vi "acc_gyro_sync_logger.vi"() -> ()   [LabVIEW 2012]
uses:
  acc_gyro_sync_data.ctl
  <vilib>/Instr/_visa.llb/VISA Configure Serial Port (Instr).vi
panel:
  out "Error":u32(graph)
  out "rate":dbl[unit]
  out "errors":i32
  out "trigger":bool
  in  "frame rate (fps)":dbl=100.0
  in  "Baud rate":u32=57600
  out "Accelerometer":waveform(dbl)[](graph)
  out "Gyro":waveform(dbl)[](graph)
  in  "accel range (m/s2)":dbl(ring)=2.0 items=["2"=2.0, "4"=4.0, "8"=8.0, "16"=16.0]
  in  "gyro range (deg/s)":dbl(ring)=250.0 items=["250"=250.0, "500"=500.0, "1000"=1000.0, "2000"=2000.0]
  in  "Serial port":refnum<visa-resource-name>="COM3"
  in  "stop":bool
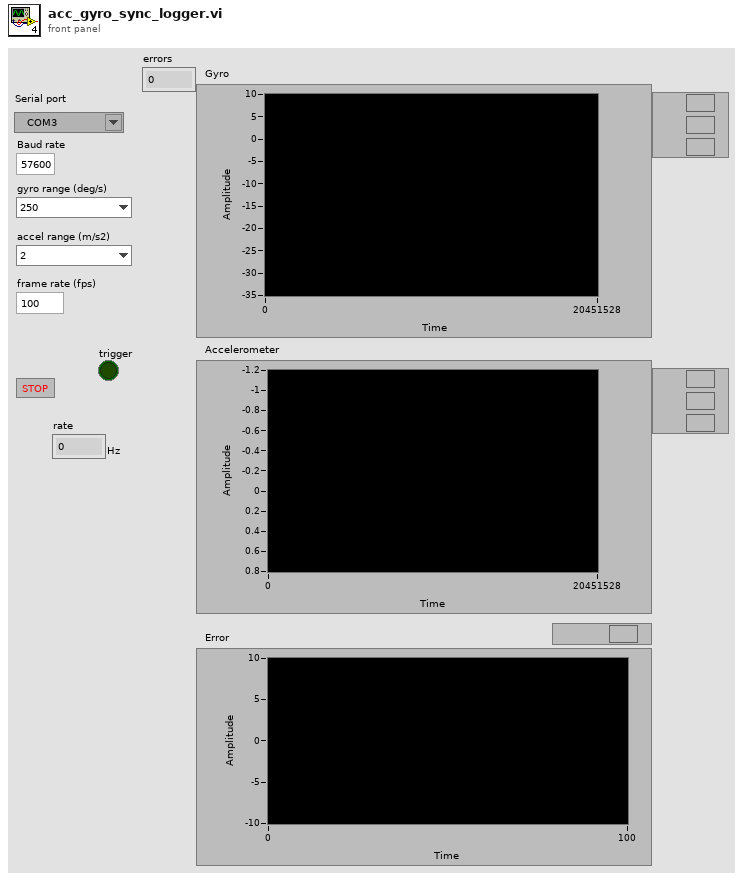
[diagram p1: front panel]
types:
  T1 = typedef "acc_gyro_sync_data.ctl" = cluster{"microsec":u32, "istrigger":u8, "gyro_x":dbl, "gyro_y":dbl, "gyro_z":dbl, "acc_x":dbl, "acc_y":dbl, "acc_z":dbl, "error":u32}
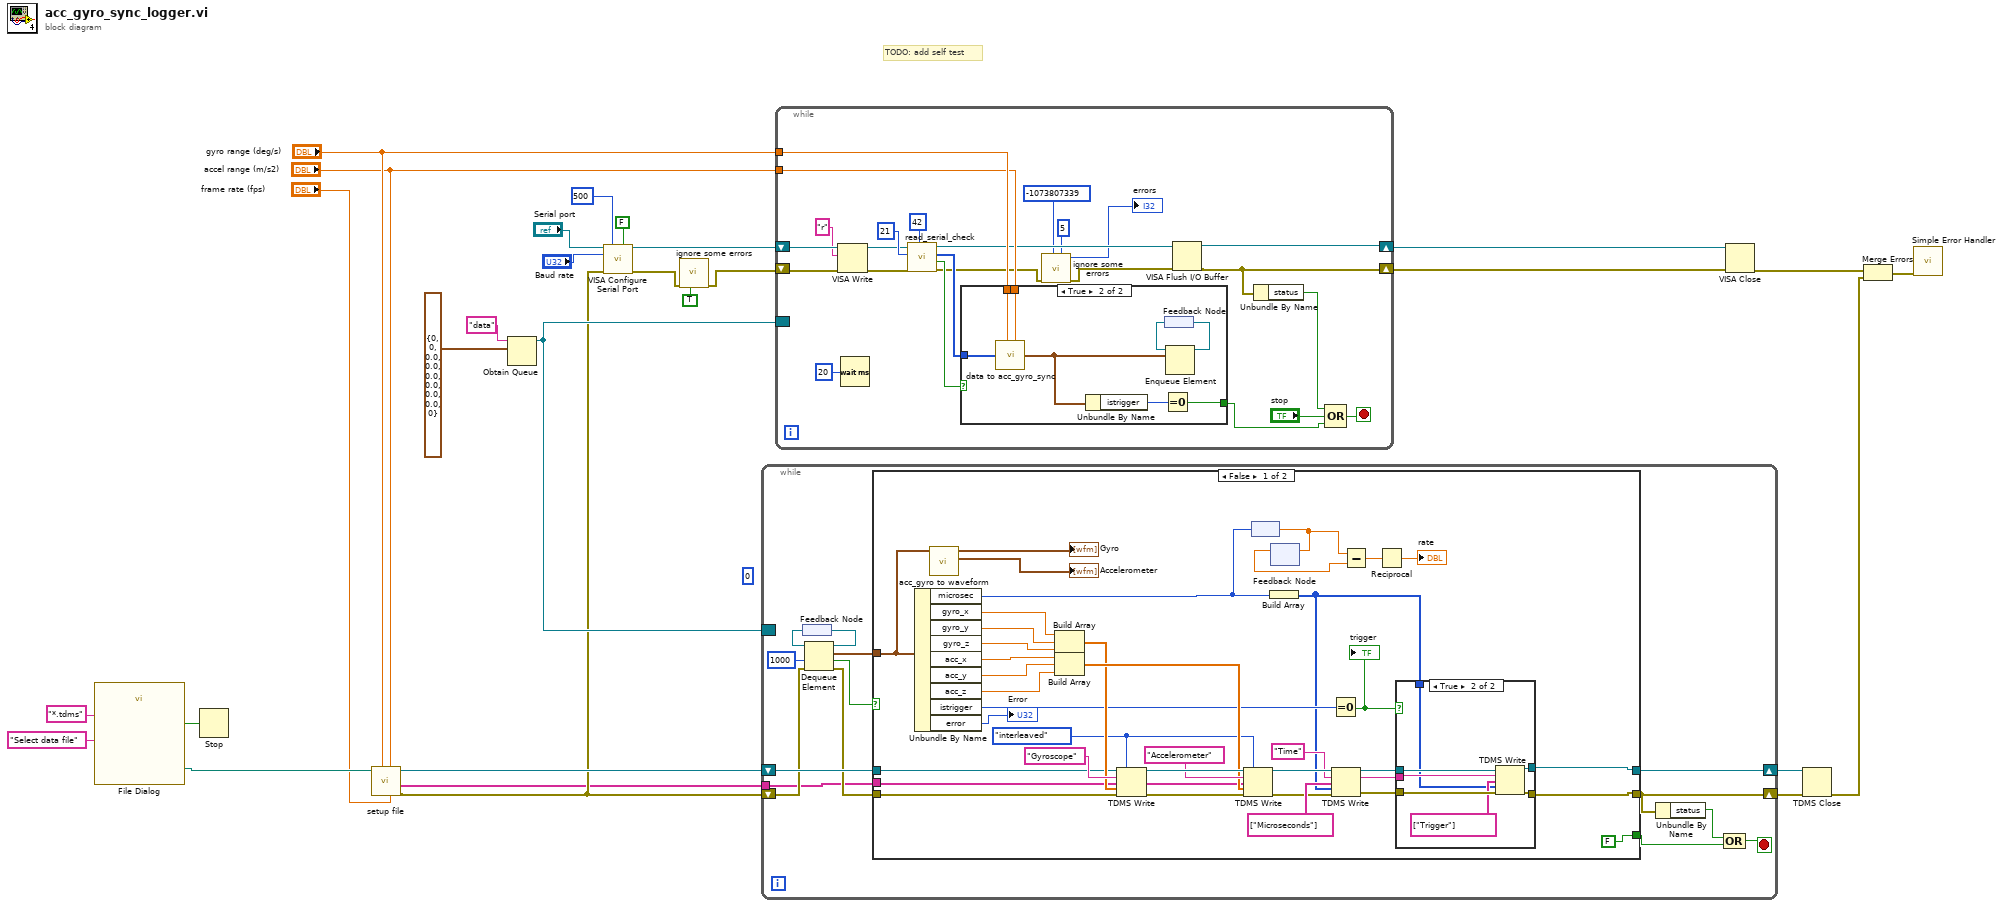
[diagram p0: block diagram]
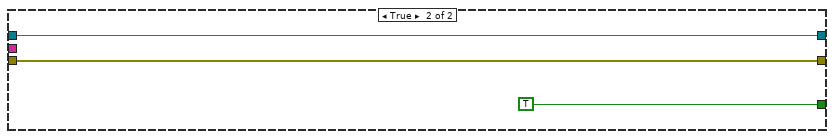
[diagram p3: hidden frame]
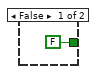
[diagram p4: hidden frame]
diagram:
  (unwired) u64 0 ("milliseconds")
  # "TODO: add self test"
  n1 = call "File Dialog"("prompt"="Select data file", "pattern (all files)"="*.tdms") -> ("selected path"=w21:path, "cancelled"=w20:bool)  [unwired: 10 in, 2 out]
  n2 = Stop(stop? (T)=w20) -> ()
  n3 = call "setup file.vi"("frame rate"="frame rate (fps)", "accel range"="accel range (m/s2)", "gyro range"="gyro range (deg/s)", "selected path"=w21) -> ("error out"=w10:errorcluster, "channel names"=w7:string[], "tdms file out"=w11:refnum<k34>)  [unwired: 5 in]
  n4 = Obtain Queue(name (unnamed)="data", element data type=T1 {"microsec"=0, "istrigger"=0, "gyro_x"=0.0, "gyro_y"=0.0, "gyro_z"=0.0, "acc_x"=0.0, "acc_y"=0.0, "acc_z"=0.0, "error"=0} ("acc gyro data")) -> (queue out=w19:refnum<queue>)  [unwired: 3 in, 2 out]
  n5 = call-poly "VISA Configure Serial Port"("VISA resource name"="Serial port", "timeout (10sec)"=u32 500, "Enable Termination\nChar (T)"=FALSE ("Enable Termination\nChar (T)"), "baud rate (9600)"="Baud rate", "error in (no error)"=w10) -> ("VISA resource name out"=w5:refnum<visa-resource-name>, "error out"=w4:errorcluster)  [unwired: 9 in]
  n6 = call "ignore some errors.vi"("reset"=TRUE, "error in"=w4) -> ("error out"=w3:errorcluster)  [unwired: 8 in, 1 out]
  n7 = while {
    border: w19 -> [_]
    shift-right: [w33] -> w16
    shift-left: w10 -> [w36]
    shift-right: [w38] -> w15
    shift-left: w11 -> [w39]
    tunnel: w7 -> [w29]
    stop <- w30 stop-if-true
    n8 = feedback #1() -> (w42:refnum<queue>)
    n9 = Dequeue Element(queue=w42, timeout in ms (-1)=1000, error in (no error)=w36) -> (queue out=w41:refnum<queue>, element=w40:T1, timed out?=w34:bool, error out=w35:errorcluster)
    n10 = feedback-in #1(w41) -> ()
    n11 = case shown="False" w34 {
      tunnel: w40 -> [w67 _]
      tunnel: [w50 w91] -> w33
      tunnel: w39 -> [w58 w92]
      tunnel: [w51 w92] -> w38
      tunnel: w35 -> [w59 w91]
      tunnel: [FALSE TRUE] -> w31
      tunnel: w29 -> [w64 _]
      frame False {
        w57 = enum16{"decimated", "interleaved"}."interleaved" ("data layout (0:decimated)")
        n12 = Unbundle By Name(w67) -> ("microsec"=w48:u32, "gyro_x"=w81:dbl, "gyro_y"=w80:dbl, "gyro_z"=w79:dbl, "acc_x"=w78:dbl, "acc_y"=w77:dbl, "acc_z"=w76:dbl, "istrigger"=w52:u8, "error"=→"Error":u32)
        n13 = call "acc_gyro to waveform.vi"("acc gyro data"=w67) -> ("accel plot"=→"Accelerometer":waveform(dbl)[], "gyro plot"=→"Gyro":waveform(dbl)[])  [unwired: 9 in]
        n14 = Build Array(w81, w80, w79) -> (w68:dbl[])
        n15 = Build Array(w78, w77, w76) -> (w71:dbl[])
        n16 = TDMS Write(0:w58, 1:w57, 5:"Gyroscope" ("group name (Untitled)"), 7:w64, 9:w68, 11:w59) -> (4:w74:refnum<k34>, 8:w63:string[], 15:w73:errorcluster)  [unwired: 1 out]
        n17 = TDMS Write(0:w74, 1:w57, 5:"Accelerometer" ("group name (Untitled)"), 7:w63, 9:w71, 11:w73) -> (4:w62:refnum<k34>, 15:w61:errorcluster)  [unwired: 2 out]
        n18 = node(w48) -> (w47:dbl[unit])
        n19 = Build Array(w48) -> (w49:u32[])
        n20 = feedback-in #2(w47) -> ()
        n21 = feedback #2() -> (w46:dbl[unit])  [unwired: 1 in]
        n22 = Equal To 0?(x=w52) -> (x = 0?=w56:bool)
        "trigger" <- w56
        n23 = TDMS Write(0:w62, 5:"Time" ("group name (Untitled)"), 7:string[] ["Microseconds"] ("channel name(s) in (Untitled)"), 9:w49, 11:w61) -> (4:w55:refnum<k34>, 6:w54:string, 15:w53:errorcluster)  [unwired: 1 in, 1 out]
        n24 = Subtract(x=w47, y=w46) -> (x-y=w45:dbl[unit])
        n25 = Reciprocal(x=w45) -> (1/x=→"rate":dbl[unit])
        n26 = case shown="True" w56 {
          tunnel: w55 -> [w83 w90]
          tunnel: w54 -> [_ w86]
          tunnel: w53 -> [w82 w89]
          tunnel: w49 -> [_ w84]
          tunnel: [w83 w88] -> w51
          tunnel: [w82 w87] -> w50
          frame False {
          }
          frame True {
            n27 = TDMS Write(0:w90, 5:w86, 7:string[] ["Trigger"] ("channel name(s) in (Untitled)"), 9:w84, 11:w89) -> (4:w88:refnum<k34>, 15:w87:errorcluster)  [unwired: 1 in, 2 out]
          }
        }
      }
      frame True {
      }
    }
    n28 = Unbundle By Name(w33) -> ("status"=w32:bool)
    n29 = Compound Arithmetic op=OR(w32, w31) -> (w30:bool)
  }
  n30 = while {
    tunnel: "gyro range (deg/s)" -> [w112]
    tunnel: "accel range (m/s2)" -> [w111]
    border: w19 -> [_]
    shift-right: [w101] -> w18
    shift-left: w3 -> [w108]
    shift-right: [w102] -> w17
    shift-left: w5 -> [w117]
    stop <- w105 stop-if-true
    n31 = VISA Write(VISA resource name=w117, write buffer="r", error in (no error)=w108) -> (VISA resource name out=w110:refnum<visa-resource-name>, error out=w107:errorcluster)  [unwired: 1 out]
    n32 = Wait (ms)(milliseconds to wait=u32 20) -> ()  [unwired: 1 out]
    n33 = call "read_serial_check.vi"("checkval"=u8 42, "error in (no error)"=w107, "byte count"=u32 21, "VISA resource name"=w110) -> ("error out"=w100:errorcluster, "good"=w114:bool, "data"=w113:u8[], "VISA resource out"=w103:refnum<visa-resource-name>)  [unwired: 4 in]
    n34 = case shown="True" w114 {
      tunnel: w113 -> [_ w126]
      tunnel: w112 -> [_ w125]
      tunnel: w111 -> [_ w124]
      tunnel: [FALSE w119] -> w94
      frame False {
      }
      frame True {
        n35 = call "data to acc_gyro_sync.vi"("byte array"=w126, "gyro range (deg/s)"=w125, "accel range (m/s2)"=w124) -> ("acc gyro data"=w121:T1)
        n36 = Unbundle By Name(w121) -> ("istrigger"=w120:u8)
        n37 = Equal To 0?(x=w120) -> (x = 0?=w119:bool)
        n38 = feedback #3() -> (w122:refnum<queue>)
        n39 = Enqueue Element(queue=w122, element=w121) -> (queue out=w123:refnum<queue>)  [unwired: 2 in, 2 out]
        n40 = feedback-in #3(w123) -> ()
      }
    }
    n41 = call "ignore some errors.vi"("max errors"=5, "error code"=-1073807339, "error in"=w100) -> ("error out"=w99:errorcluster, "errors"=→"errors":i32)  [unwired: 7 in]
    n42 = VISA Flush I/O Buffer(VISA resource name=w103, error in (no error)=w99) -> (VISA resource name out=w102:refnum<visa-resource-name>, error out=w101:errorcluster)  [unwired: 1 in]
    n43 = Unbundle By Name(w101) -> ("status"=w104:bool)
    n44 = Compound Arithmetic op=OR(w104, "stop", w94) -> (w105:bool)
  }
  n45 = VISA Close(VISA resource name=w17, error in (no error)=w18) -> (error out=w14:errorcluster)
  n46 = TDMS Close(8:w16, 11:w15) -> (0:w13:errorcluster)  [unwired: 1 out]
  n47 = Merge Errors(w14, w13) -> (w12:errorcluster)
  n48 = call <vilib>:"Simple Error Handler.vi"("error in (no error)"=w12) -> ()  [unwired: 4 in, 5 out]
